vi "ackNoPermCMD.vi"(8 "error in (no error)":errorcluster, 9 "rejectedReason":string, 10 "CommandValue":T1=enum."disable", 11 "Model in":refnum<class "Model.lvclass">) -> (0 "error out":errorcluster, 3 "Model out":refnum<class "Model.lvclass">)   [LabVIEW 2016, in "Model.lvclass"]
uses:
  Model.lvclass
  Typedefs/CommandValue.ctl
  Model.lvclass/Model.ctl
  PubSubDataEvent/PubSubDataEvent.lvclass/PubSubDataEvent.ctl
  Typedefs/SEDSpectrometerTypedefs.lvlib
  PubSubDataEvent/PubSubDataEvent.lvclass
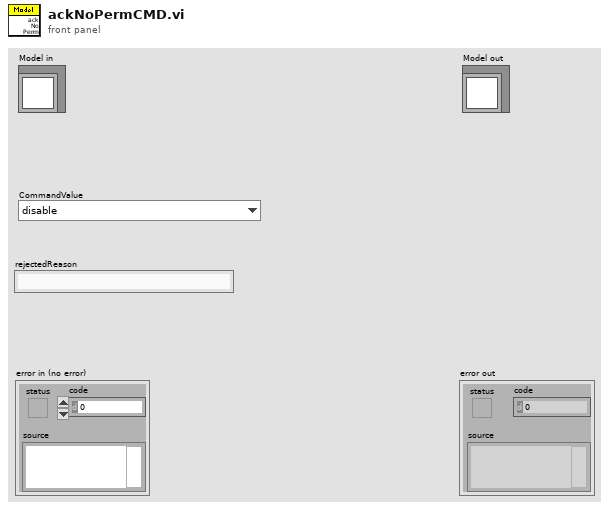
[diagram p1: front panel]
types:
  T1 = typedef "SEDSpectrometerTypedefs.lvlib/CommandValue.ctl" = enum16{"clearError", "disable", "enable", "exit", "GoToStandby", "OnHeartbeat", "OnIncomingMessagingError", "OnInterrupt", "start", "captureSpectImage", "setSpectTempSetpoint", "stopImageCapture"}
  T2 = cluster{"error":i32, "result":string, "ack":i32, "cmdSeqNum":i32, "CommandValue":T1}
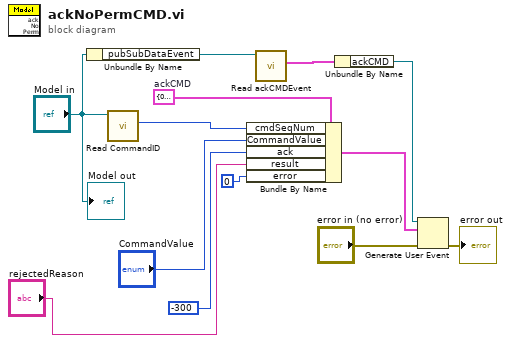
[diagram p0: block diagram]
diagram:
  w13 = T2 {"error"=0, "result"="", "ack"=0, "cmdSeqNum"=0, "CommandValue"=enum."disable"}  # ackCMD
  n1 = Unbundle By Name("Model in") -> ("pubSubDataEvent"=w12:refnum<class "PubSubDataEvent.lvclass">)
  n2 = call-dynamic "Read CommandID.vi"("Model in"="Model in") -> ("CommandID"=w5:i32)  [unwired: 8 in, 2 out]
  n3 = Bundle By Name(cluster=w13, "cmdSeqNum"=w5, "CommandValue"="CommandValue", "ack"=-300, "result"="rejectedReason", "error"=0) -> (w9:T2)
  n4 = call "Read ackCMDEvent.vi"("PubSubDataEvent in"=w12) -> ("ackCMDEvent"=w11:cluster{"ackCMD":refnum<user-event>})  [unwired: 8 in, 2 out]
  n5 = Unbundle By Name(w11) -> ("ackCMD"=w10:refnum<user-event>)
  n6 = Generate User Event(user event=w10, event data cluster=w9, error in="error in (no error)") -> (error out=→"error out":errorcluster)  [unwired: 1 in, 1 out]
  "Model out" <- "Model in"
